vi "Host - Get ECAT IOVs.vi"(0 "ECAT Slave in":refnum<k21>="ni.var.io:/", 11 "error in (no error)":errorcluster) -> (4 "ECAT Slave out":refnum<k21>="ni.var.io:/", 6 "UDV Container":refnum<k21>[](array[refnum]), 8 "ECAT Variablenobjekt":refnum<k21>[](array[refnum]), 10 "All Mods":refnum<k21>[](array[refnum]), 15 "error IO":errorcluster)   [LabVIEW 2016, in "Scan Engine Custom Device.lvlib"]
uses:
  Scan Engine Custom Device.lvlib
  <resource>/objmgr/IndComECAT.rc
  <resource>/objmgr/ni.var.rc
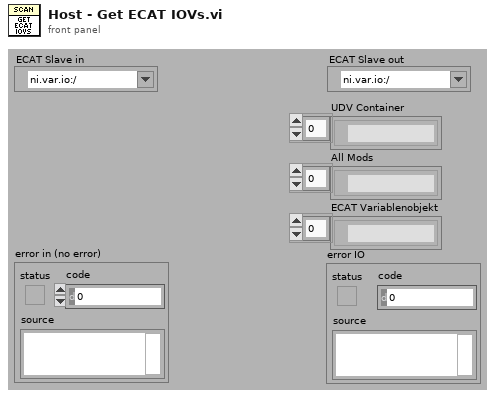
[diagram p1: front panel]
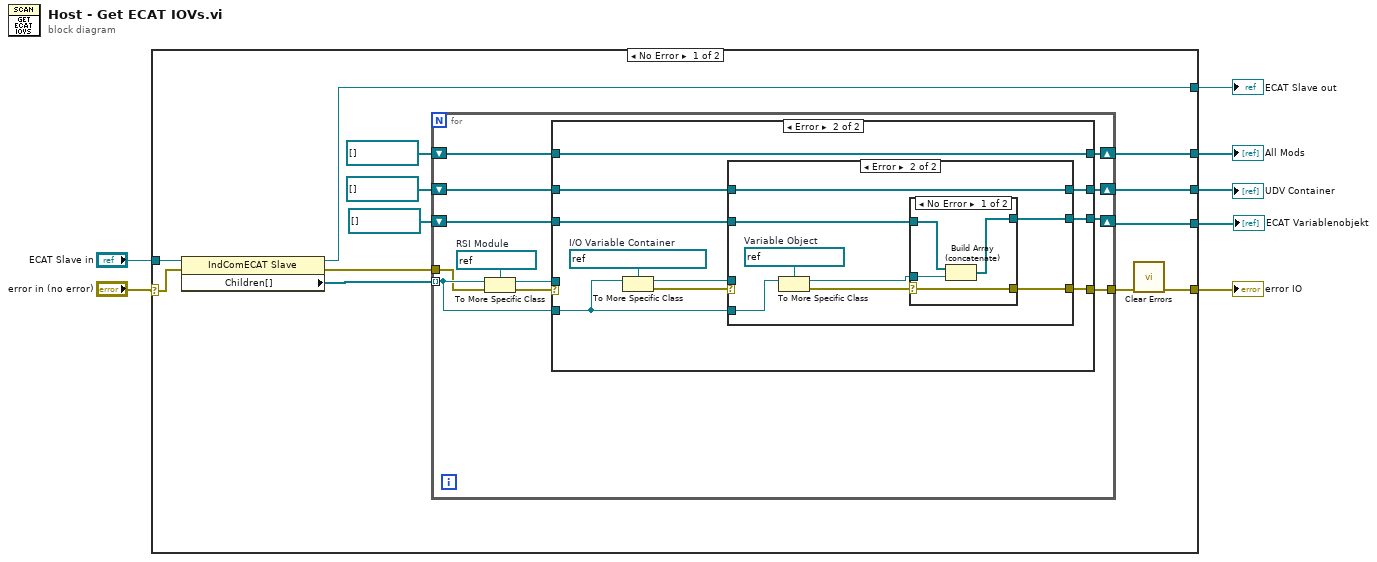
[diagram p0: block diagram]
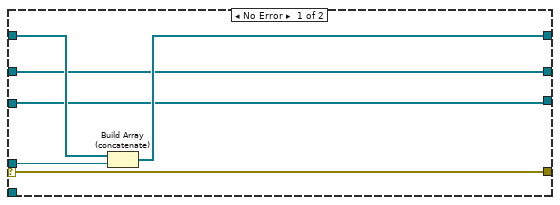
[diagram p2: hidden frame]
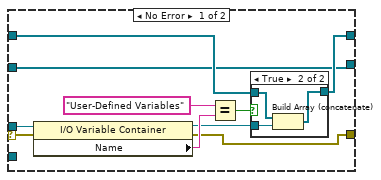
[diagram p3: hidden frame]
diagram:
  n1 = case shown="No Error" "error in (no error)" {
    selector: "error in (no error)" -> [w17 w78]
    tunnel: [w20 w78] -> w7
    tunnel: [w13 _] -> w3
    tunnel: "ECAT Slave in" -> [w19 w77]
    tunnel: [w18 w77] -> w5
    tunnel: [w10 _] -> w2
    tunnel: [w8 _] -> w1
    frame No Error {
      n2 = property class="IndComECAT Slave"(reference=w19, error in=w17) -> (reference out=w18:refnum<k21>, error out=w14:errorcluster, "Children[]"=w15:refnum<k21>[])
      n3 = for {
        tunnel: w15 -> [w24] mode=indexing
        tunnel: w14 -> [w23]
        shift-right: [w31] -> w13
        shift-left: refnum<k21>[] [] -> [w30]
        tunnel: [w29] -> w12
        shift-right: [w25] -> w10
        shift-left: refnum<k21>[] [] -> [w26]
        shift-right: [w21] -> w8
        shift-left: refnum<k21>[] [] -> [w22]
        w32 = refnum<k21> refnum  # RSI Module
        n4 = To More Specific Class(target class=w32, reference=w24, error in=w23) -> (specific class reference=w27:refnum<k21>, error out=w28:errorcluster)
        n5 = case shown="Error" w28 {
          selector: w28 -> [w34 _]
          tunnel: w27 -> [w35 _]
          tunnel: [w38 w48] -> w31
          tunnel: w30 -> [w37 w48]
          tunnel: [w34 w42] -> w29
          tunnel: w26 -> [w36 w44]
          tunnel: [w36 w43] -> w25
          tunnel: w24 -> [_ w41]
          tunnel: w22 -> [w33 w40]
          tunnel: [w33 w39] -> w21
          frame No Error {
            n6 = Build Array (concatenate)(w37, w35) -> (w38:refnum<k21>[])
          }
          frame Error {
            w47 = refnum<k21> refnum  # I/O Variable Container
            n7 = To More Specific Class(target class=w47, reference=w41) -> (specific class reference=w45:refnum<k21>, error out=w46:errorcluster)  [unwired: 1 in]
            n8 = case shown="Error" w46 {
              selector: w46 -> [w58 _]
              tunnel: [w52 w64] -> w43
              tunnel: w45 -> [w57 _]
              tunnel: [w51 w63] -> w42
              tunnel: w44 -> [w50 w64]
              tunnel: w41 -> [_ w69]
              tunnel: w40 -> [w49 w66]
              tunnel: [w49 w65] -> w39
              frame No Error {
                n9 = property class="I/O Variable Container"(reference=w57, error in=w58) -> (reference out=w53:refnum<k21>, error out=w51:errorcluster, "Name"=w56:string)
                n10 = Equal?(x="User-Defined Variables", y=w56) -> (x = y?=w54:bool)
                n11 = case shown="True" w54 {
                  tunnel: w53 -> [_ w61]
                  tunnel: w50 -> [w59 w62]
                  tunnel: [w59 w60] -> w52
                  frame False {
                  }
                  frame True {
                    n12 = Build Array (concatenate)(w62, w61) -> (w60:refnum<k21>[])
                  }
                }
              }
              frame Error {
                w70 = refnum<k21> refnum  # Variable Object
                n13 = To More Specific Class(target class=w70, reference=w69) -> (specific class reference=w67:refnum<k21>, error out=w68:errorcluster)  [unwired: 1 in]
                n14 = case shown="No Error" w68 {
                  selector: w68 -> [w71 w76]
                  tunnel: [w74 w75] -> w65
                  tunnel: w67 -> [w73 _]
                  tunnel: w66 -> [w72 w75]
                  tunnel: [w71 w76] -> w63
                  frame No Error {
                    n15 = Build Array (concatenate)(w72, w73) -> (w74:refnum<k21>[])
                  }
                  frame Error {
                  }
                }
              }
            }
          }
        }
      }
      n16 = call <vilib>:"Clear Errors.vi"("error in (no error)"=w12) -> ("error out"=w20:errorcluster)  [unwired: 5 in, 1 out]
    }
    frame Error {
    }
  }
  "error IO" <- w7
  "ECAT Slave out" <- w5
  "All Mods" <- w3
  "UDV Container" <- w2
  "ECAT Variablenobjekt" <- w1
